vi "ControlFunction.vi"(8 "error in (no error)":errorcluster, 11 "RobotLift in":refnum<class "RobotLift.lvclass">) -> (0 "error out":errorcluster, 3 "RobotLift out":refnum<class "RobotLift.lvclass">)   [LabVIEW 2017, in "RobotLift.lvclass"]
uses:
  RobotLift.lvclass
  SubsystemData/RobotLiftData/RobotLiftData.lvclass
  R:/Documents/github/FRC4080/2018-robot-main/SubsystemData/SubsystemData.lvclass
  RobotLift.lvclass/RobotLift.ctl
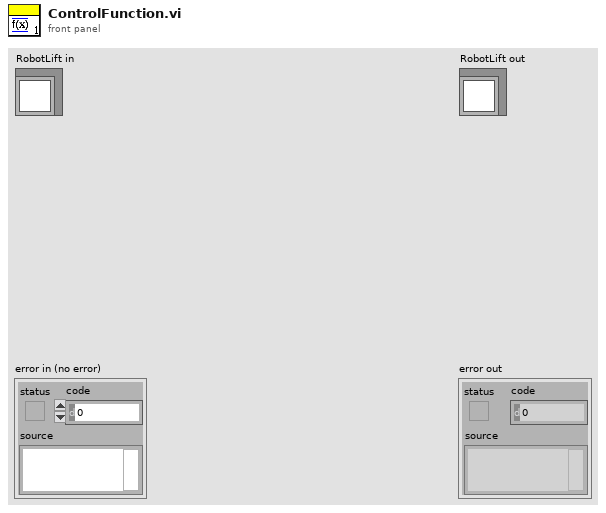
[diagram p1: front panel]
types:
  T1 = typedef "RobotLiftData.lvclass/RobotLiftCommand.ctl" = cluster{"Left Lift":cluster{"Up":bool, "Down":bool}, "Right Lift":cluster{"Up":bool, "Down":bool}, "Release Ramps":bool, "Mode":T2}
  T2 = typedef "RobotSubsystem.lvclass/RunMode.ctl" = enum16{"Auto", "Teleop", "Disabled"}
  T3 = typedef "RobotLiftData.lvclass/RobotLiftOutput.ctl" = cluster{"LeftRobotLiftSetting":dbl, "RightRobotLiftSetting":dbl, "RampReleaseSetting":bool}
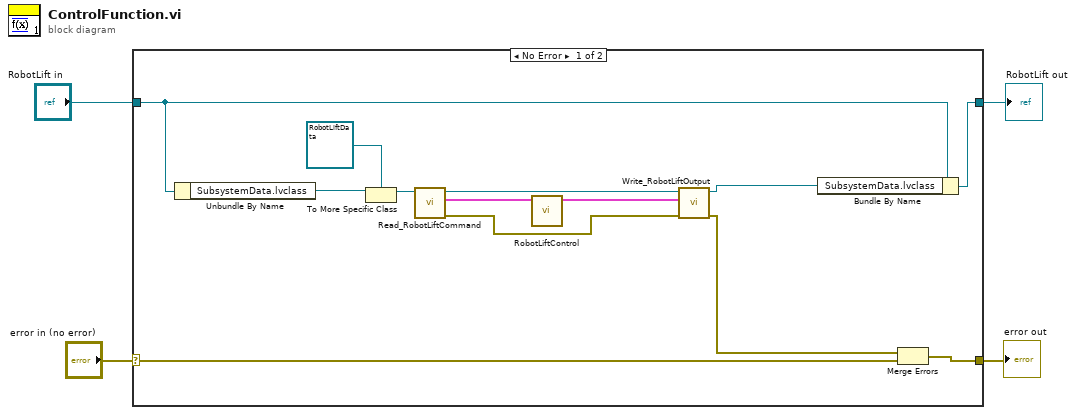
[diagram p0: block diagram]
diagram:
  n1 = case shown="No Error" "error in (no error)" {
    selector: "error in (no error)" -> [w17 w18]
    tunnel: [w12 w18] -> w3
    tunnel: "RobotLift in" -> [w15 w19]
    tunnel: [w16 w19] -> w1
    frame No Error {
      n2 = Unbundle By Name(w15) -> ("SubsystemData.lvclass"=w14:refnum<class "SubsystemData.lvclass">)
      n3 = To More Specific Class(target class=refnum<class "RobotLiftData.lvclass"> refnum ("RobotLiftData.lvclass"), reference=w14) -> (specific class reference=w11:refnum<class "RobotLiftData.lvclass">)  [unwired: 1 in, 1 out]
      n4 = call-dynamic "Read_RobotLiftCommand.vi"("RobotLiftData in"=w11) -> ("error out"=w7:errorcluster, "Robot Lift Command"=w10:T1, "RobotLiftData out"=w8:refnum<class "RobotLiftData.lvclass">)  [unwired: 8 in]
      n5 = call "RobotLiftControl.vi"("Robot Lift Command"=w10) -> ("RobotLiftOutput out"=w9:T3)  [unwired: 10 in]
      n6 = call-dynamic "Write_RobotLiftOutput.vi"("error in (no error)"=w7, "RobotLiftOutput"=w9, "RobotLiftData in"=w8) -> ("error out"=w6:errorcluster, "RobotLiftData out"=w5:refnum<class "RobotLiftData.lvclass">)  [unwired: 7 in]
      n7 = Bundle By Name(cluster=w15, "SubsystemData.lvclass"=w5) -> (w16:refnum<class "RobotLift.lvclass">)
      n8 = Merge Errors(w6, w17) -> (w12:errorcluster)
    }
    frame Error {
    }
  }
  "error out" <- w3
  "RobotLift out" <- w1
